vi "SENSe.vi"(8 "Error in (no error)":errorcluster, 9 "Range":string="Auto", 10 "Function":enum16{"SENSe", "SENSe Query"}(ring)=enum."SENSe Query", 11 "VISA resource":refnum<visa-resource-name>) -> (0 "Error out":errorcluster, 1 "Auto":bool, 2 "Range out":string, 3 "Dup VISA resource":refnum<visa-resource-name>)   [LabVIEW 2010]
doc: "Copyright (c) 2012 Metrolab Technology SA, Plan-les-Ouates, Geneva, Switzerland\nSets the measurement range, or gets the currently selected range. Note that it can be very useful to get the currently selected range after performing an auto-ranging measurement."
panel:
  # "SENSe"
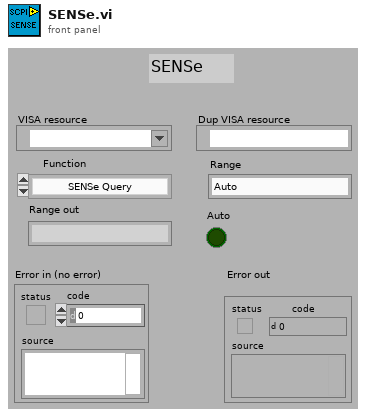
[diagram p1: front panel]
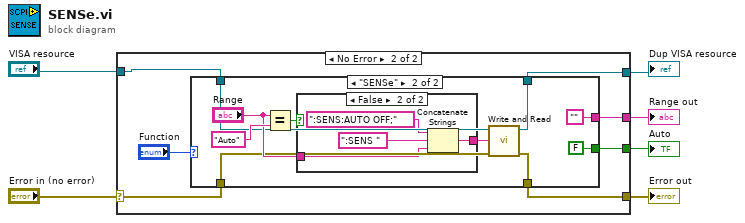
[diagram p0: block diagram]
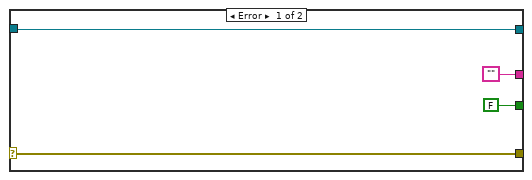
[diagram p2: hidden frame]
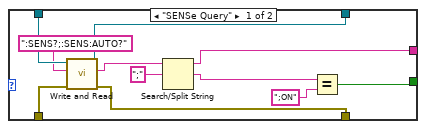
[diagram p3: hidden frame]
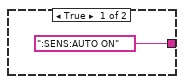
[diagram p4: hidden frame]
diagram:
  n1 = case shown="No Error" "Error in (no error)" {
    selector: "Error in (no error)" -> [w9 w15]
    tunnel: "VISA resource" -> [w10 w16]
    tunnel: [w10 w14] -> w4
    tunnel: [w9 w13] -> w6
    tunnel: ["" ("Response") w12] -> w2
    tunnel: [FALSE w11] -> w1
    frame Error {
    }
    frame No Error {
      n2 = case shown="\"SENSe\"" "Function" {
        tunnel: w16 -> [w27 w34]
        tunnel: w15 -> [w28 w33]
        tunnel: [w24 w32] -> w14
        tunnel: [w25 w31] -> w13
        tunnel: [w21 ""] -> w12
        tunnel: [w20 FALSE] -> w11
        frame "SENSe Query" {
          n3 = call "Write and Read.vi"("Error in (no error)"=w28, "Command"=":SENS?;:SENS:AUTO?" (":SENSe[:FLUX][:RANGe]:AUTO ON"), "VISA resource"=w27) -> ("Error out"=w25:errorcluster, "Response"=w22:string, "Dup VISA resource"=w24:refnum<visa-resource-name>)  [unwired: 4 in, 2 out]
          n4 = Search/Split String(string=w22, search string/char (-)=";") -> (substring before match=w21:string, match + rest of string=w19:string)  [unwired: 1 in, 1 out]
          n5 = Equal?(x=w19, y=";ON") -> (x = y?=w20:bool)
        }
        frame "SENSe" {
          n6 = Equal?(x="Range", y="Auto") -> (x = y?=w37:bool)
          n7 = case shown="False" w37 {
            tunnel: [":SENS:AUTO ON" (":SENSe[:FLUX][:RANGe]:AUTO ON") w43] -> w35
            tunnel: "Range" -> [_ w40]
            frame True {
            }
            frame False {
              n8 = Concatenate Strings(":SENS:AUTO OFF;" (":SENSe[:FLUX][:RANGe][:UPPer]"), ":SENS " ("string"), w40) -> (w43:string)
            }
          }
          n9 = call "Write and Read.vi"("Error in (no error)"=w33, "Command"=w35, "VISA resource"=w34) -> ("Error out"=w31:errorcluster, "Dup VISA resource"=w32:refnum<visa-resource-name>)  [unwired: 4 in, 3 out]
        }
      }
    }
  }
  "Error out" <- w6
  "Dup VISA resource" <- w4
  "Range out" <- w2
  "Auto" <- w1
